vi "Dual Display activation.vi"() -> ()   [LabVIEW 2016, in "Generic Digital Multi Meter.lvlib" / "Tektronix DMM4020.lvlib" / "Tektronix DMM4020.lvclass"]
uses:
  Tektronix DMM4020.lvclass
  <instrlib>/Tektronix DMM4020/Tektronix DMM4020.lvlib
panel:
  out "error in (no error)":errorcluster
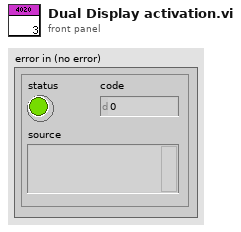
[diagram p1: front panel]
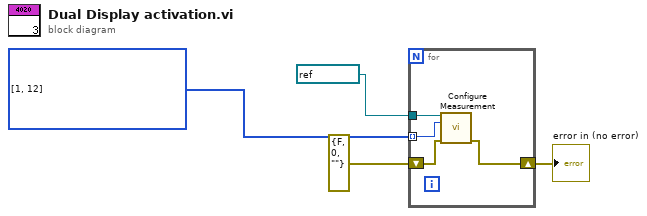
[diagram p0: block diagram]
diagram:
  w3 = u16[] [1, 12] items=["DC Volts", "AC Volts", "DC Current", "AC Current", "2-Wire Resistance", "4-Wire Resistance", "Frequency", "AC and DC rms Current", "AC and DC rms Volts", "Continuity", "Diode", "AC Current 2", "AC Volts 2"]
  n1 = for {
    tunnel: refnum<visa-resource-name> "COM7" ("VISA Address") -> [w8]
    tunnel: w3 -> [w7] mode=indexing
    shift-right: [w5] -> w1
    shift-left: errorcluster {"status"=FALSE, "code"=0, "source"=""} ("error in (no error)") -> [w6]
    n2 = call <instrlib>:"Configure Measurement.vi"("VISA resource name"=w8, "Measurement Function (0: DC Volts)"=w7, "error in (no error)"=w6) -> ("error out"=w5:errorcluster)  [unwired: 11 in, 1 out]
  }
  "error in (no error)" <- w1
